vi "SIM BDF factor accelerator.vi"(8 "current timestep index":i32, 10 "step size":dbl, 11 "BDF data":T1) -> (0 "error":bool, 3 "BDF data out":T1)   [LabVIEW 2020]
uses:
  SIM BDF data.ctl
  SIM Factored Matrix.ctl
  SIM BDF stages.ctl
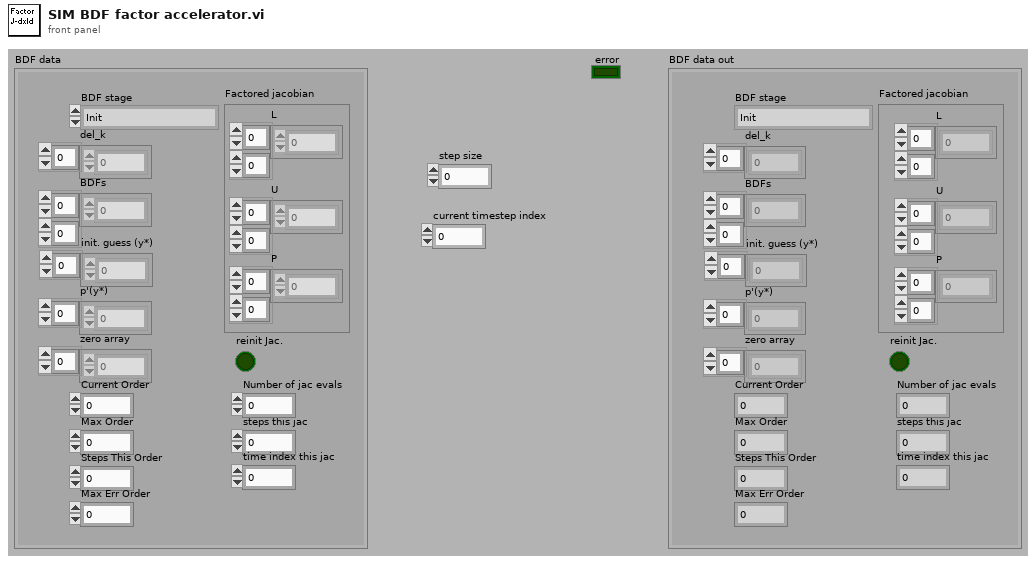
[diagram p1: front panel]
types:
  T1 = typedef "SIM BDF data.ctl" = cluster{"BDFs":dbl[][], "init. guess (y*)":dbl[], "p'(y*)":dbl[], "Factored jacobian":T2, "zero array":dbl[], "reinit Jac.":bool, "BDF stage":T3, "steps this jac":i32, "time index this jac":i32, "Number of jac evals":i32, "del_k":dbl[], "Current Order":i32, "Max Order":i32, "Steps This Order":i32, "Max Err Order":i32}
  T2 = typedef "SIM Factored Matrix.ctl" = cluster{"L":dbl[][], "U":dbl[][], "P":i32[][]}
  T3 = typedef "SIM BDF stages.ctl" = enum16{"Init", "Initial Guess", "Compute Jacobian", "Newton Iteration", "Eval Error", "Choose StepSize", "Reset BDFs"}
  T4 = typedef "NI_Matrix.lvlib/RealMatrix.ctl" = dbl[][]
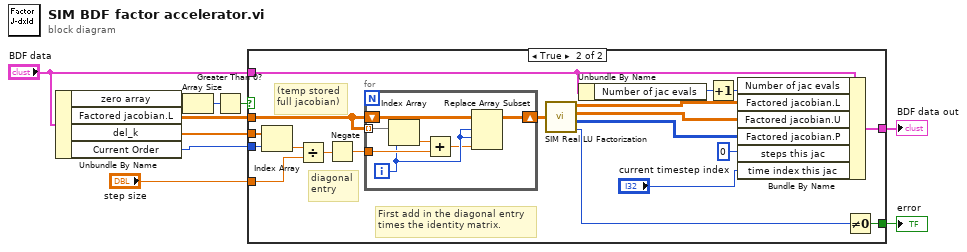
[diagram p0: block diagram]
diagram:
  n1 = Unbundle By Name("BDF data") -> ("zero array"=w3:dbl[], "Factored jacobian.L"=w4:dbl[][], "del_k"=w7:dbl[], "Current Order"=w8:i32)
  n2 = Array Size(array=w3) -> (size(s)=w2:i32)
  n3 = Greater Than 0?(x=w2) -> (x > 0?=w1:bool)
  n4 = case shown="True" w1 {
    tunnel: [w11 w30] -> w10
    tunnel: [_ w24] -> w9
    tunnel: w8 -> [_ w22]
    tunnel: w7 -> [_ w21]
    tunnel: "step size" -> [_ w20]
    tunnel: "BDF data" -> [w11 w18]
    tunnel: w4 -> [_ w17]
    frame False {
    }
    frame True {
      # "diagonal\nentry"
      # "(temp stored\nfull jacobian)"
      # "First add in the diagonal entry\ntimes the identity matrix."
      n5 = Index Array(array=w21, index=w22) -> (element=w23:dbl)
      n6 = Divide(x=w23, y=w20) -> (x/y=w19:dbl)
      n7 = Negate(x=w19) -> (-x=w25:dbl)
      n8 = for {
        shift-right: [w33] -> w16
        shift-left: w17 -> [w34]
        tunnel: w25 -> [w35]
        tunnel: w17 -> [w37] mode=indexing
        i -> [w32]
        n9 = Index Array(array=w37, index=w32) -> (element=w36:dbl)
        n10 = Add(x=w36, y=w35) -> (x+y=w31:dbl)
        n11 = Replace Array Subset(array=w34, new element=w31, index (row)=w32, index (col)=w32) -> (w33:dbl[][])
      }
      n12 = call "SIM Real LU Factorization.vi"("A"=w16) -> ("L"=w15:T4, "U"=w14:T4, "P"=w13:i32[][], "error"=w12:i32)
      n13 = Unbundle By Name(w18) -> ("Number of jac evals"=w27:i32)
      n14 = Increment(x=w27) -> (x+1=w26:i32)
      n15 = Bundle By Name(cluster=w18, "Number of jac evals"=w26, "Factored jacobian.L"=w15, "Factored jacobian.U"=w14, "Factored jacobian.P"=w13, "steps this jac"=0, "time index this jac"="current timestep index") -> (w30:T1)
      n16 = Not Equal To 0?(x=w12) -> (x != 0?=w24:bool)
    }
  }
  "error" <- w9
  "BDF data out" <- w10
